vi "ch_filter_test1.vi"() -> ()   [LabVIEW 2021]
panel:
  in  "filter rate (+2)":u16
  in  "Numeric":i32
  out "Waveform Chart":dbl(graph)
  in  "stop":bool
  in  "s":bool
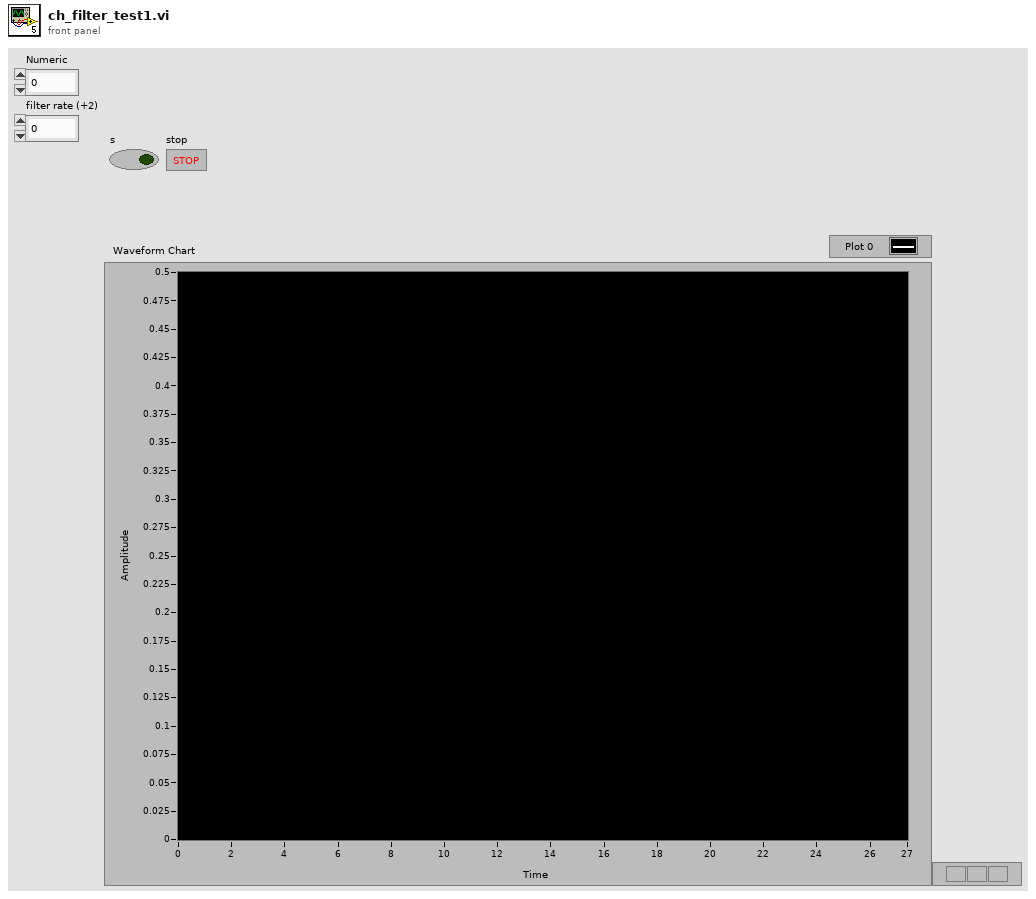
[diagram p1: front panel]
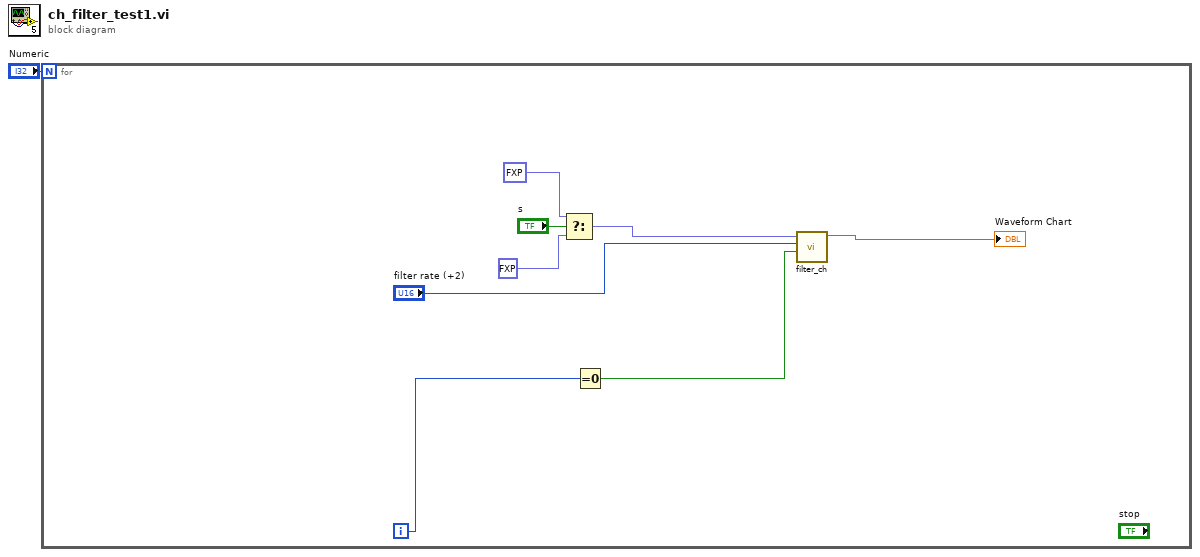
[diagram p0: block diagram]
diagram:
  n1 = for {
    N: "Numeric" -> [_]
    i -> [w3]
    n2 = Select(t=fxp<+/-,16,1> 0.5 ("input data"), s="s", f=fxp<+/-,16,1> 0.0 ("input data")) -> (s? t:f=w5:fxp<+/-,16,1>)
    n3 = Equal To 0?(x=w3) -> (x = 0?=w2:bool)
    n4 = call "filter_ch.vi"("reset"=w2, "filter rate"="filter rate (+2)", "filter in"=w5) -> ("filter out"=→"Waveform Chart":fxp<+/-,16,1>)  [unwired: 8 in]
  }
